vi "Intersection With Crosswalks.vi"() -> ()   [LabVIEW 2023]
uses:
  <extravilib>/ChannelInstances/One Element Stream-u16/Read With Abort.vi
  <extravilib>/ChannelInstances/One Element Stream-bool/Instantiate.vi
  <extravilib>/ChannelInstances/One Element Stream-u16/Instantiate.vi
  <extravilib>/ChannelInstances/One Element Stream-u16/EndpointRead.vi
  <extravilib>/ChannelInstances/One Element Stream-u16.lvlib
  <extravilib>/ChannelInstances/One Element Stream-bool.lvlib
panel:
  out "ped":u16(ring)=2
  out "ped":u16(ring)
  out "light":u16(ring)=2
  out "light":u16(ring)
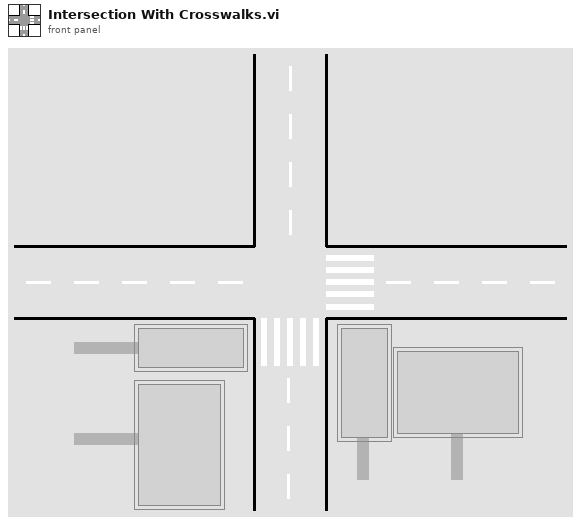
[diagram p1: front panel]
types:
  T1 = typedef "One Element Stream-bool.lvlib/)Channel.ctl" = refnum<queue>
  T2 = typedef "One Element Stream-u16.lvlib/)Channel.ctl" = refnum<queue>
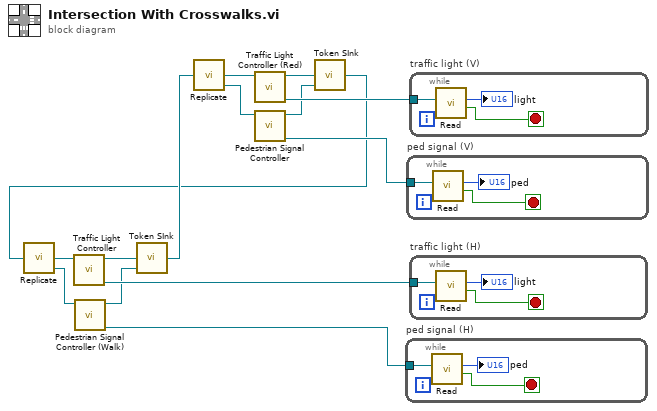
[diagram p0: block diagram]
diagram:
  n1 = call <extravilib>:"Replicate.vi"("one element stream"=w2) -> ("one element stream copy 1"=w9:T1, "one element stream copy 2"=w8:T1)  [unwired: 7 in]
  n2 = call "Traffic Light Controller.vi"("peds stopped"=w9) -> ("traffic light"=w14:T2, "cars stopped"=w6:T1)  [unwired: 5 in]
  n3 = call "Pedestrian Signal Controller (Walk).vi"("cars stopped"=w8) -> ("ped signal"=w7:T2, "peds stopped"=w4:T1)  [unwired: 9 in]
  n4 = call "Token SInk.vi"("token 1"=w6, "token 2"=w4) -> ("token out"=w5:T1)  [unwired: 7 in]
  n5 = call <extravilib>:"Replicate.vi"("one element stream"=w5) -> ("one element stream copy 1"=w11:T1, "one element stream copy 2"=w10:T1)  [unwired: 7 in]
  n6 = call "Traffic Light Controller (Red).vi"("peds stopped"=w11) -> ("traffic light"=w13:T2, "cars stopped"=w3:T1)  [unwired: 5 in]
  n7 = call "Pedestrian Signal Controller.vi"("cars stopped"=w10) -> ("ped signal"=w12:T2, "peds stopped"=w1:T1)  [unwired: 9 in]
  n8 = call "Token SInk.vi"("token 1"=w3, "token 2"=w1) -> ("token out"=w2:T1)  [unwired: 7 in]
  n9 = while "ped signal (H)" {
    tunnel: w7 -> [w17]
    stop <- w16 stop-if-true
    n10 = call <extravilib>:"Read.vi"("channel"=w17) -> ("last element?"=w16:bool, "element"=→"ped":u16)  [unwired: 7 in, 2 out]
  }
  n11 = while "ped signal (V)" {
    tunnel: w12 -> [w20]
    stop <- w19 stop-if-true
    n12 = call <extravilib>:"Read.vi"("channel"=w20) -> ("last element?"=w19:bool, "element"=→"ped":u16)  [unwired: 7 in, 2 out]
  }
  n13 = while "traffic light (V)" {
    tunnel: w13 -> [w23]
    stop <- w22 stop-if-true
    n14 = call <extravilib>:"Read.vi"("channel"=w23) -> ("last element?"=w22:bool, "element"=→"light":u16)  [unwired: 7 in, 2 out]
  }
  n15 = while "traffic light (H)" {
    tunnel: w14 -> [w26]
    stop <- w25 stop-if-true
    n16 = call <extravilib>:"Read.vi"("channel"=w26) -> ("last element?"=w25:bool, "element"=→"light":u16)  [unwired: 7 in, 2 out]
  }
